vi "RH_DCPower_Initialize.vi"(8 "error in":errorcluster, 11 "resource name":refnum<k15> caption="DCPower Resource Name") -> (0 "error out":errorcluster, 3 "DCPower Session Out":refnum<k15>)   [LabVIEW 2023, in "ResourceHandling.lvlib"]
doc: "Initializes the resource by setting default values"
uses:
  ResourceHandling.lvlib
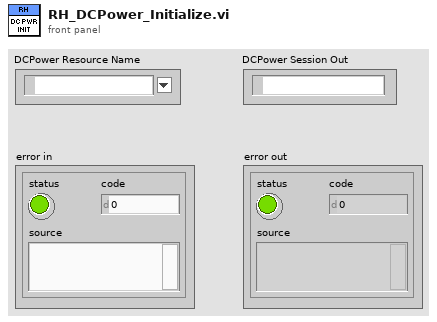
[diagram p1: front panel]
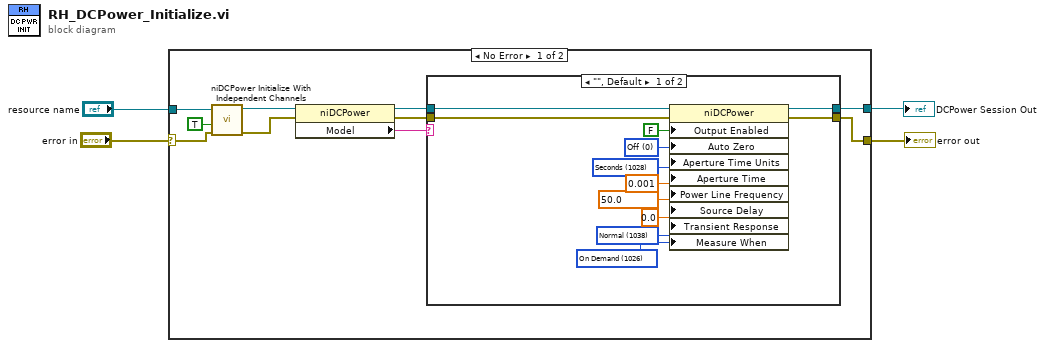
[diagram p0: block diagram]
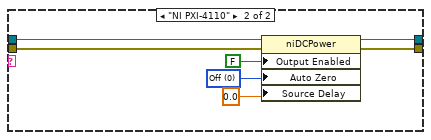
[diagram p2: hidden frame]
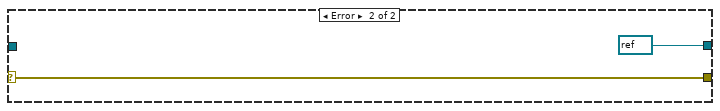
[diagram p3: hidden frame]
diagram:
  n1 = case shown="No Error" "error in" {
    selector: "error in" -> [w5 w35]
    tunnel: "resource name" -> [w8 _]
    tunnel: [w7 refnum<k15> refnum ("instrument handle out")] -> w3
    tunnel: [w6 w35] -> w2
    frame No Error {
      n2 = call <instrlib>:"niDCPower Initialize With Independent Channels.vi"("error in (no error)"=w5, "reset (false)"=TRUE, "resource name"=w8) -> ("error out"=w12:errorcluster, "instrument handle out"=w10:refnum<k15>)  [unwired: 7 in]
      n3 = property class="niDCPower"(reference=w10, error in=w12) -> (reference out=w9:refnum<k15>, error out=w11:errorcluster, "Model"=w13:string)
      n4 = case shown="\"\", Default" w13 {
        tunnel: w9 -> [w26 w33]
        tunnel: w11 -> [w25 w32]
        tunnel: [w18 w28] -> w6
        tunnel: [w17 w27] -> w7
        frame "", Default {
          w15 = 1026 items=["Automatically after Source Complete"=1025, "On Demand"=1026, "On Measure Trigger"=1027] ("Measurement:Advanced:Measure When")
          w16 = 1038 items=["Slow"=1041, "Normal"=1038, "Fast"=1039, "Custom"=1042] ("Source:Transient Response")
          w20 = 50.0 items=["60 Hertz"=60.0, "50 Hertz"=50.0] ("Measurement:Power Line Frequency")
          w22 = 1028 items=["Seconds"=1028, "Power Line Cycles"=1029] ("Measurement:Aperture Time Units")
          w23 = 0 items=["Off"=0, "Once"=1024, "On"=1] ("Measurement:Auto Zero")
          n5 = property class="niDCPower"(reference=w26, error in=w25, "Output Enabled"=FALSE ("Source:Output Enabled"), "Auto Zero"=w23, "Aperture Time Units"=w22, "Aperture Time"=0.001 ("Measurement:Aperture Time"), "Power Line Frequency"=w20, "Source Delay"=0.0 ("Source:Advanced:Source Delay"), "Transient Response"=w16, "Measure When"=w15) -> (reference out=w17:refnum<k15>, error out=w18:errorcluster)
        }
        frame "NI PXI-4110" {
          w30 = 0 items=["Off"=0, "Once"=1024, "On"=1] ("Measurement:Auto Zero")
          n6 = property class="niDCPower"(reference=w33, error in=w32, "Output Enabled"=FALSE ("Source:Output Enabled"), "Auto Zero"=w30, "Source Delay"=0.0 ("Source:Advanced:Source Delay")) -> (reference out=w27:refnum<k15>, error out=w28:errorcluster)
        }
      }
    }
    frame Error {
    }
  }
  "DCPower Session Out" <- w3
  "error out" <- w2
